vi "keccak.remain.helper.8.block_size.vi"(9 "HT_DATA.Valid":bool, 10 "HT_DATA.Data":u64, 11 "Variables":T2={"hash.input_size"=0, "hash.bits"=0, "state.next"=enum."Wait.for.Start", "state.after_next"=enum."Wait.for.Start", "read.i"=0, "read.block_i"=0, "hash.block_words"=0, "hash.block_size"=0, "keccak.i"=0, "state[25]"=[0, 0, 0, 0, 0, 0, 0, 0, 0, 0, 0, 0, 0, 0, 0, 0, 0, 0, 0, 0, 0, 0, 0, 0, 0], "HT_PARMS.Valid"=FALSE, "HT_PARMS.Data"=0, "Read.HT_PARMS"=FALSE, "HT_DATA.Valid"=FALSE, "HT_DATA.Data"=0, "Read.HT_DATA"=FALSE, "TH_RESULTS.Valid"=FALSE, "TH_RESULTS.Data"=0, "TH_RESULTS.Ready"=FALSE}) -> (0 "state.next":T1=enum."Keccak", 1 "state[25] out":u64[](array[numeric]), 2 "Continue?":bool, 3 "Valid":bool, 4 "read.block_i":u16)   [LabVIEW 2021]
uses:
  Users/johns/OneDrive/Documents/LabVIEW Data/Untitled Project 2/CLIP/keccak.variables.ctl
  Users/johns/OneDrive/Documents/LabVIEW Data/Untitled Project 2/CLIP/keccak.states.ctl
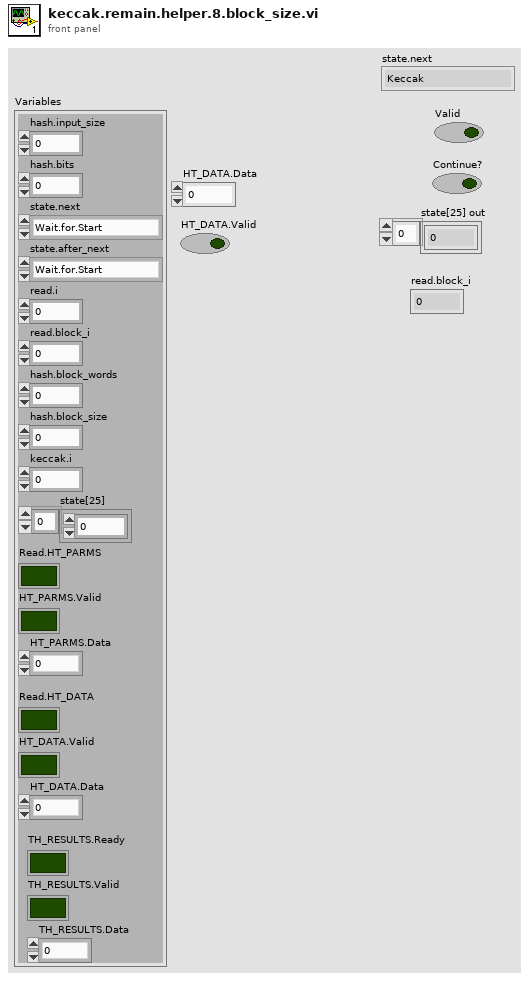
[diagram p1: front panel]
types:
  T1 = typedef "keccak.states.ctl" = enum8{"Wait.for.Start", "Read.Blocks", "Read.Remainder", "Keccak", "Send.Result"}
  T2 = typedef "keccak.variables.ctl" = cluster{"hash.input_size":u16, "hash.bits":u16, "state.next":T1, "state.after_next":T1, "read.i":u16, "read.block_i":u16, "hash.block_words":u16, "hash.block_size":u16, "keccak.i":u16, "state[25]":u64[], "HT_PARMS.Valid":bool, "HT_PARMS.Data":u64, "Read.HT_PARMS":bool, "HT_DATA.Valid":bool, "HT_DATA.Data":u64, "Read.HT_DATA":bool, "TH_RESULTS.Valid":bool, "TH_RESULTS.Data":u64, "TH_RESULTS.Ready":bool}
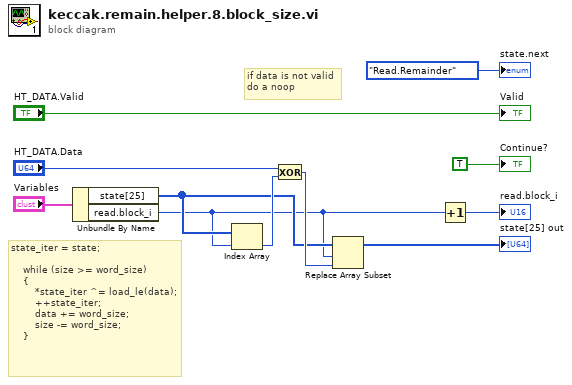
[diagram p0: block diagram]
diagram:
  # "if data is not valid\ndo a noop"
  # "state_iter = state;\n\n    while (size >= word_size)\n    {\n        *state_iter ^= load_le(data);\n        ++state_iter;\n        data += word_size;\n        size -= word_size;\n    }"
  n1 = Unbundle By Name("Variables") -> ("state[25]"=w7:u64[], "read.block_i"=w2:u16)
  n2 = Index Array(array=w7, index=w2) -> (element=w9:u64)
  n3 = Exclusive Or(1:w9, 2:"HT_DATA.Data") -> (0:w10:u64)
  n4 = Replace Array Subset(array=w7, new element=w10, index=w2) -> (→"state[25] out":u64[])
  n5 = Increment(x=w2) -> (x+1=→"read.block_i":u16)
  "Valid" <- "HT_DATA.Valid"
  "Continue?" <- TRUE ("Continue?")
  "state.next" <- keccak.states."Read.Remainder" ("state.next")
